vi "Clear Attacked.vi"(11 "Array in":T1[][](array[typedef])) -> (3 "Array out":T1[][](array[typedef]))   [LabVIEW 2015, in "SB SubVIs.lvlib"]
uses:
  SB SubVIs.lvlib
  Type Defs/Square Cluster.ctl
  Square/Square.lvclass
  Globals.vi
  Type Defs/SB Type Defs.lvlib
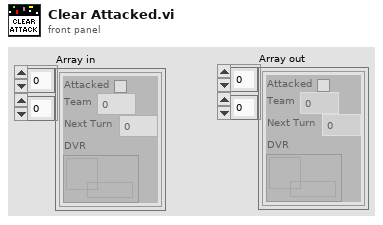
[diagram p1: front panel]
types:
  T1 = typedef "SB Type Defs.lvlib/Square Cluster.ctl" = cluster{"Attacked":bool, "Team":i32, "Next Turn":i32, "DVR":refnum<data-value>}
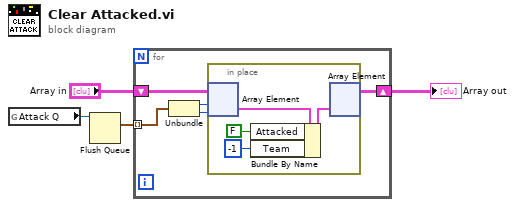
[diagram p0: block diagram]
diagram:
  n1 = global read "Globals.vi" "Attack Q"() -> (w2:refnum<queue>)
  n2 = Flush Queue(queue=w2) -> (remaining elements=w1:cluster{"Row":i32, "Column":i32}[])  [unwired: 1 in, 2 out]
  n3 = for {
    shift-right: [w8] -> w4
    shift-left: "Array in" -> [w9]
    tunnel: w1 -> [w7] mode=indexing
    n4 = Unbundle(w7) -> ("Row"=w6:i32, "Column"=w5:i32)
    n5 = in-place {
      n6 = in-place-array #1(w9, w6, w5) -> (w12:T1)
      n7 = Bundle By Name(cluster=w12, "Attacked"=FALSE ("Attacked?"), "Team"=-1) -> (w11:T1)
      n8 = in-place-array #1(w11) -> (w8:T1[][])  [unwired: 2 out]
    }
  }
  "Array out" <- w4
